vi "Add Result.vi"(8 "error in (no error)":errorcluster, 9 "TestStand Result":T1, 10 "Sequence Context In":refnum<k7>) -> (0 "error out":errorcluster)   [LabVIEW 2020, in "Astemes_CSVReportPlugin.lvlib" / "Report Generator.lvlib"]
uses:
  Report Generator.lvlib
  Test Result Handler/TestStand Result Handler.lvclass
  Astemes_CSVReportGenerator/TSContext Configuration/TSContext Configuration.lvclass
  Private/Reference.vi
  C:/git/astemes-excel-report-teststand-plugin/source/Astemes_CSVReportGenerator/TSContext Configuration/TSContext Configuration.lvclass
  C:/git/astemes-excel-report-teststand-plugin/source/Astemes_CSVReportGenerator/Configuration/Configuration.lvclass
  Test Result Handler/TestStand Result.ctl
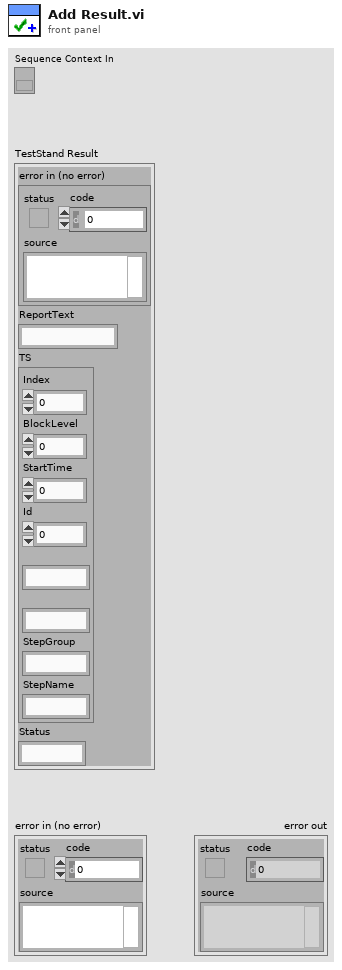
[diagram p1: front panel]
types:
  T1 = typedef "Astemes_CSVReportPlugin.lvlib/TestStand Result Handler.lvclass/TestStand Result.ctl" = cluster{"error in (no error)":errorcluster, "ReportText":string, "TS":cluster{"Index":i32, "BlockLevel":i32, "StartTime":dbl, "Id":i32, "StepType":string, "StepID":string, "StepGroup":string, "StepName":string}, "Status":string}
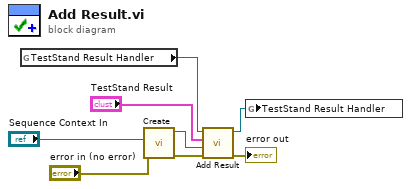
[diagram p0: block diagram]
diagram:
  n1 = global read "Reference.vi" "TestStand Result Handler"() -> (w3:refnum<class "TestStand Result Handler.lvclass">)
  n2 = call "Create.vi"("error in (no error)"="error in (no error)", "Sequence Context In"="Sequence Context In") -> ("error out"=w4:errorcluster, "TSContext Configuration"=w5:refnum<class "TSContext Configuration.lvclass">)  [unwired: 8 in]
  n3 = call "Add Result.vi"("error in (no error)"=w4, "Sequenc Context"=w5, "TestStand Result"="TestStand Result", "TestStand Result Handler In"=w3) -> ("error out"=→"error out":errorcluster, "TestStand Result Handler Out"=w2:refnum<class "TestStand Result Handler.lvclass">)  [unwired: 6 in]
  n4 = global write "Reference.vi" "TestStand Result Handler"(w2) -> ()
